vi "Insert At DataArray.vi"(8 "error in":errorcluster, 9 "index":i32, 10 "Rows":string[][](array[string]), 11 "DataGridView in":refnum<class "DataGridView.lvclass">) -> (0 "error out":errorcluster, 3 "DataGridView out":refnum<class "DataGridView.lvclass">)   [LabVIEW 2016, in "DataGrid.lvlib" / "DataGridView.lvclass"]
uses:
  <userlib>/LabVIEWdotNetDataGrid/source/DataGridView/DataGridView.lvclass
  <userlib>/LabVIEWdotNetDataGrid/source/DataGridView/DataGridView.lvclass/DataGridView.ctl
  System.Windows.Forms
  <userlib>/LabVIEWdotNetDataGrid/source/DataTable/Insert Rows At (String).vi
  <userlib>/LabVIEWdotNetDataGrid/source/DataTable/DataTable.lvclass
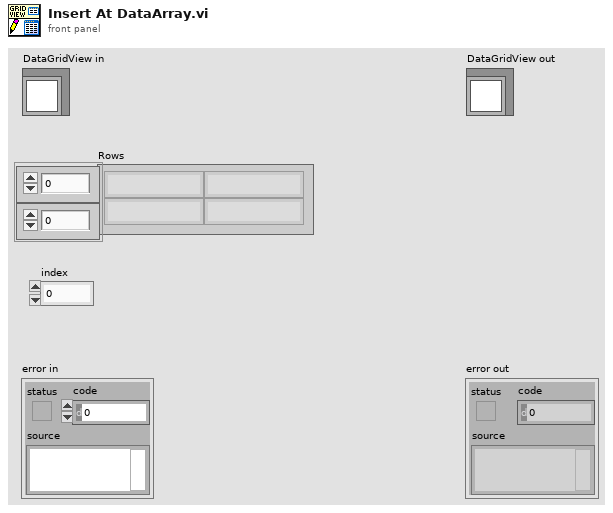
[diagram p1: front panel]
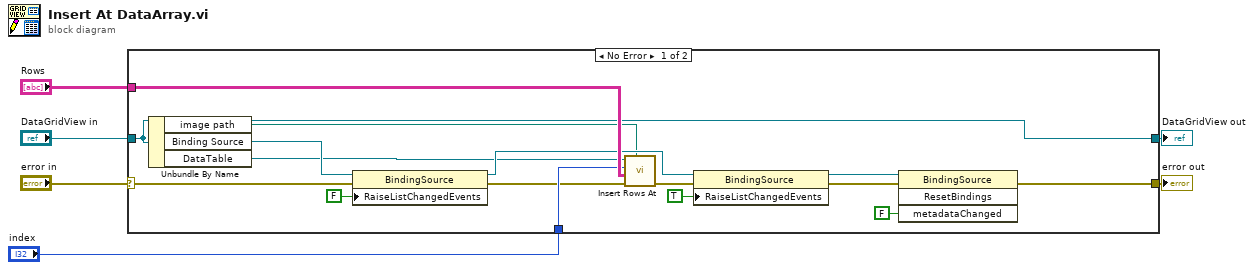
[diagram p0: block diagram]
diagram:
  n1 = case shown="No Error" "error in" {
    selector: "error in" -> [w18 w23]
    tunnel: [w8 w23] -> w5
    tunnel: [w21 w24] -> w3
    tunnel: "DataGridView in" -> [w21 w24]
    tunnel: "Rows" -> [w22 _]
    tunnel: "index" -> [w12 _]
    frame No Error {
      n2 = Unbundle By Name(w21) -> ("image path"=w11:path, "Binding Source"=w20:refnum<k24>, "DataTable"=w13:refnum<class "DataTable.lvclass">)
      n3 = property class="BindingSource"(reference=w20, error in=w18, "RaiseListChangedEvents"=FALSE) -> (reference out=w19:refnum<k24>, error out=w10:errorcluster)
      n4 = call-poly <userlib>:"Insert Rows At.vi"("image path"=w11, "error in (no error)"=w10, "String Data"=w22, "index"=w12, "DataTable in"=w13) -> ("error out"=w7:errorcluster)  [unwired: 5 in, 1 out]
      n5 = property class="BindingSource"(reference=w19, error in=w7, "RaiseListChangedEvents"=TRUE) -> (reference out=w16:refnum<k24>, error out=w9:errorcluster)
      n6 = invoke class="BindingSource" method="ResetBindings"(reference=w16, error in=w9, "metadataChanged"=FALSE) -> (error out=w8:errorcluster)  [unwired: 1 in, 3 out]
    }
    frame Error {
    }
  }
  "error out" <- w5
  "DataGridView out" <- w3
